vi "命令字符串选择.vi"(11 "枚举":enum16{"获取SN", "获取门禁状态", "远程开门", "更新权限"}(ring)) -> (3 "字符串":string)   [LabVIEW 2016, in "环境动力监测库.lvlib" / "智能门禁监测.lvlib"]
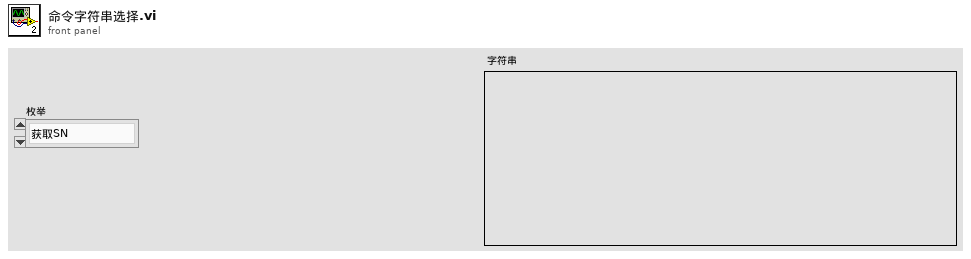
[diagram p1: front panel]
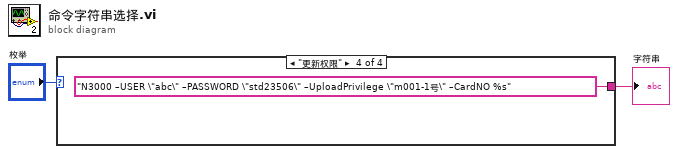
[diagram p0: block diagram]
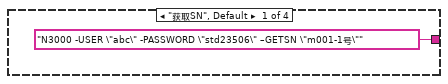
[diagram p2: hidden frame]
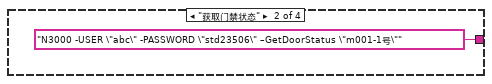
[diagram p3: hidden frame]
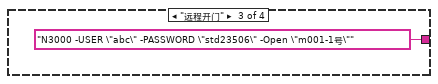
[diagram p4: hidden frame]
diagram:
  n1 = case shown="\"更新权限\"" "枚举" {
    tunnel: ["N3000 -USER \"abc\" -PASSWORD \"std23506\" –GETSN \"m001-1号\"" "N3000 -USER \"abc\" -PASSWORD \"std23506\" –GetDoorStatus \"m001-1号\"" "N3000 -USER \"abc\" -PASSWORD \"std23506\" -Open \"m001-1号\"" "N3000 –USER \"abc\" –PASSWORD \"std23506\" –UploadPrivilege \"m001-1号\" –CardNO %s"] -> w1
    frame "获取SN", Default {
    }
    frame "获取门禁状态" {
    }
    frame "远程开门" {
    }
    frame "更新权限" {
    }
  }
  "字符串" <- w1
